vi "Add Bus Status Section with Channels.vi"(8 "error in":errorcluster, 11 "custom device":T1 format="%.0x") -> (0 "error out":errorcluster, 1 "bus status channels":T1[](array[typedef]) format="%.0x", 2 "bus status section":T1 format="%.0x", 3 "custom device out":T1 format="%.0x")   [LabVIEW 2020, in "AIM MIL-STD-1553 Scripting.lvlib"]
doc: "Adds a Message Section to the specified <b>bus controller</b> using the name in <b>message name</b> and returns a reference to the added <b>message section</b>."
uses:
  AIM MIL-STD-1553 Scripting.lvlib
  <vilib>/NI VeriStand/Custom Device API/Custom Device Item Ref.ctl
  <vilib>/NI VeriStand/Custom Device API/Custom Device Channel.ctl
  <vilib>/NI VeriStand/Custom Device API/Custom Device Channel Type.ctl
  Constants.vi
  <vilib>/NI VeriStand/Custom Device API/Custom Device API.lvlib
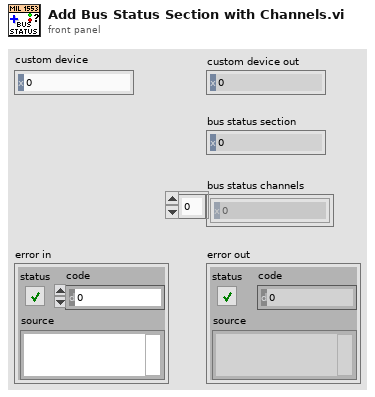
[diagram p1: front panel]
types:
  T1 = typedef "Custom Device API.lvlib/Custom Device Item Ref.ctl" = u64
  T2 = typedef "Custom Device API.lvlib/Custom Device Channel.ctl" = cluster{"Type":T3, "Units":string, "Default Value":dbl, "Faultable":bool, "Scalable":bool}
  T3 = typedef "Custom Device API.lvlib/Custom Device Channel Type.ctl" = enum16{"Input", "Output"}
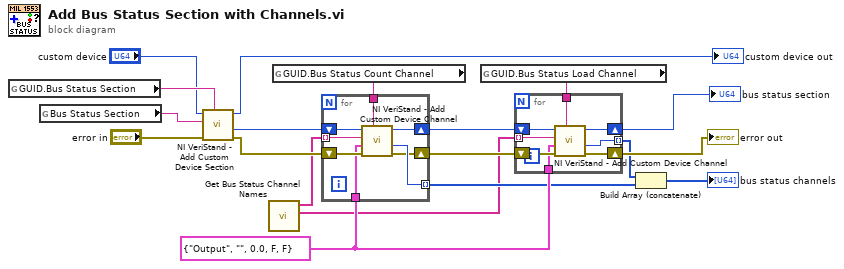
[diagram p0: block diagram]
diagram:
  w10 = T2 {"Type"=enum."Output", "Units"="", "Default Value"=0.0, "Faultable"=FALSE, "Scalable"=FALSE} ("Channel")
  n1 = global read "Constants.vi" "GUID.Bus Status Section"() -> (w19:string)
  n2 = global read "Constants.vi" "Bus Status Section"() -> (w16:string)
  n3 = call <vilib>:"NI VeriStand - Add Custom Device Section.vi"("GUID (Default Section)"=w19, "error in (no error)"="error in", "Section Name"=w16, "Parent Ref in"="custom device") -> ("error out"=w15:errorcluster, "Section Ptr"=w13:T1, "Parent Ref out"=→"custom device out":T1)  [unwired: 4 in, 1 out]
  n4 = call "Get Bus Status Channel Names.vi"() -> ("bus status loads"=w1:string[], "bus status counts"=w2:string[])  [unwired: 10 in]
  n5 = global read "Constants.vi" "GUID.Bus Status Count Channel"() -> (w14:string)
  n6 = for {
    tunnel: w2 -> [w26] mode=indexing
    tunnel: w14 -> [w25]
    tunnel: w10 -> [w23]
    shift-right: [w22] -> w11
    shift-left: w13 -> [w24]
    tunnel: [w21] -> w7 mode=indexing
    shift-right: [w20] -> w12
    shift-left: w15 -> [w27]
    n7 = call <vilib>:"NI VeriStand - Add Custom Device Channel.vi"("GUID (Default Channel)"=w25, "error in (no error)"=w27, "Channel"=w23, "Channel Name"=w26, "Parent Ref in"=w24) -> ("error out"=w20:errorcluster, "Channel Ref"=w21:T1, "Parent Ref out"=w22:T1)  [unwired: 3 in, 1 out]
  }
  n8 = global read "Constants.vi" "GUID.Bus Status Load Channel"() -> (w9:string)
  n9 = for {
    tunnel: w1 -> [w34] mode=indexing
    tunnel: w9 -> [w33]
    tunnel: w10 -> [w31]
    shift-right: [w30] -> w3
    shift-left: w11 -> [w32]
    tunnel: [w29] -> w6 mode=indexing
    shift-right: [w28] -> w8
    shift-left: w12 -> [w35]
    n10 = call <vilib>:"NI VeriStand - Add Custom Device Channel.vi"("GUID (Default Channel)"=w33, "error in (no error)"=w35, "Channel"=w31, "Channel Name"=w34, "Parent Ref in"=w32) -> ("error out"=w28:errorcluster, "Channel Ref"=w29:T1, "Parent Ref out"=w30:T1)  [unwired: 3 in, 1 out]
  }
  "error out" <- w8
  "bus status section" <- w3
  n11 = Build Array (concatenate)(w6, w7) -> (→"bus status channels":T1[])
